vi "TIFF View IFD Array.vi"(8 "error in (no error)":errorcluster, 11 "TIFF in":refnum<class "TIFF.lvclass">) -> (0 "error out":errorcluster, 3 "IFD Array":refnum<class "IFD.lvclass">[](array[class]))   [LabVIEW 2016, in "TIFF.lvclass"]
uses:
  TIFF.lvclass
  IFD/IFD.lvclass
  TIFF.lvclass/TIFF.ctl
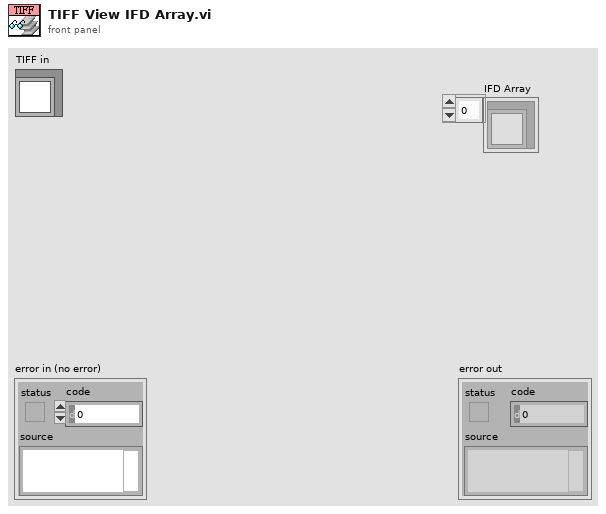
[diagram p1: front panel]
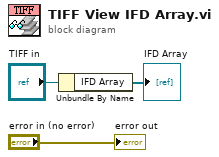
[diagram p0: block diagram]
diagram:
  n1 = Unbundle By Name("TIFF in") -> ("IFD Array"=→"IFD Array":refnum<class "IFD.lvclass">[])
  "error out" <- "error in (no error)"
